vi "Deserialize CD XML FIle.vi"(8 "Error In":errorcluster caption="error in", 11 "XML Path":path) -> (0 "Error Out":errorcluster caption="error in", 3 "Custom Device .NET Ref Out":refnum<k24>)   [LabVIEW 2015, in "VeriStand Custom Device XML Parser.lvlib"]
doc: "Deserializes the provided custom device XML file and returns a reference to the file in memory."
uses:
  NationalInstruments.VeriStand.XMLReader
  <vilib>/Utility/sysdir.llb/System Directory Type.ctl
  subVI/Config Global.vi
  VeriStand Custom Device XML Parser.lvlib
  Configuration Tool.lvlib
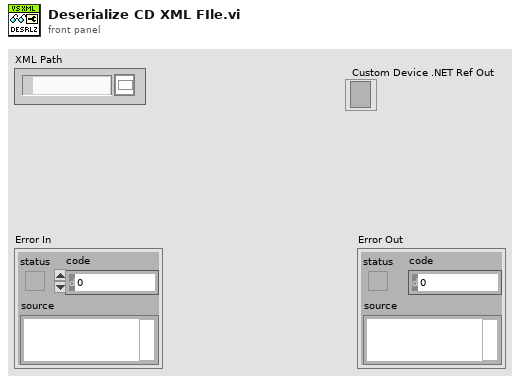
[diagram p1: front panel]
types:
  T1 = typedef "System Directory Type.ctl" = i32
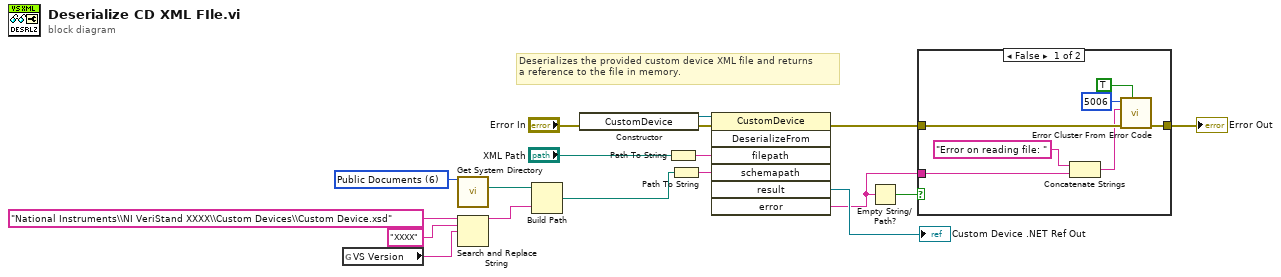
[diagram p0: block diagram]
diagram:
  w14 = T1 6 items=["User Home"=0, "User Desktop"=1, "User Documents"=2, "User Application Data"=3, "User Preferences"=4, "User Temporary"=5, "Public Documents"=6, "Public Application Data"=7, "Public Preferences"=8, "Public Cache"=13, "System Core Libraries"=9, "System Installed Libraries"=10, "Application Files"=11, "Boot Volume Root"=12] ("system directory type")
  # "Deserializes the provided custom device XML file and returns\na reference to the file in memory."
  n1 = global read "Config Global.vi" "VS Version"() -> (w8:string)
  n2 = call <vilib>:"Get System Directory.vi"("system directory type"=w14) -> ("system directory"=w13:path)  [unwired: 10 in]
  n3 = Search and Replace String(input string="National Instruments\\NI VeriStand XXXX\\Custom Devices\\Custom Device.xsd", search string="XXXX", replace string=w8) -> (result string=w7:string)  [unwired: 5 in, 3 out]
  n4 = Build Path(base path=w13, name or relative path=w7) -> (appended path=w12:path)
  n5 = constructor class="CustomDevice"(error in="Error In") -> (reference out=w16:refnum<k24>, error out=w5:errorcluster)  [unwired: 2 in, 1 out]
  n6 = Path To String(path="XML Path") -> (string=w15:string)
  n7 = Path To String(path=w12) -> (string=w11:string)
  n8 = invoke class="CustomDevice" method="DeserializeFrom"(reference=w16, error in=w5, "filepath"=w15, "schemapath"=w11) -> (error out=w2:errorcluster, "result"=→"Custom Device .NET Ref Out":refnum<k24>, "error"=w3:string)  [unwired: 3 in, 4 out]
  n9 = Empty String/Path?(string/path=w3) -> (empty?=w4:bool)
  n10 = case shown="False" w4 {
    tunnel: w3 -> [w24 _]
    tunnel: w2 -> [w23 w26]
    tunnel: [w20 w26] -> w1
    frame False {
      n11 = Concatenate Strings("Error on reading file: " ("string"), w24) -> (w21:string)
      n12 = call <vilib>:"Error Cluster From Error Code.vi"("show call chain? (False)"=TRUE, "error in (no error)"=w23, "error message (\"\")"=w21, "error code (0)"=5006) -> ("error out"=w20:errorcluster)  [unwired: 5 in]
    }
    frame True {
    }
  }
  "Error Out" <- w1
